vi "PH_Test.vi"() -> ()   [LabVIEW 8.6]
panel:
  out "Router Info":T1(array[cluster])
  out "Range":i32
  out "Resolution (ps)":i32
  out "error out":errorcluster
  out "Library Version":string="2.1"
  in  "error in (no error)":errorcluster
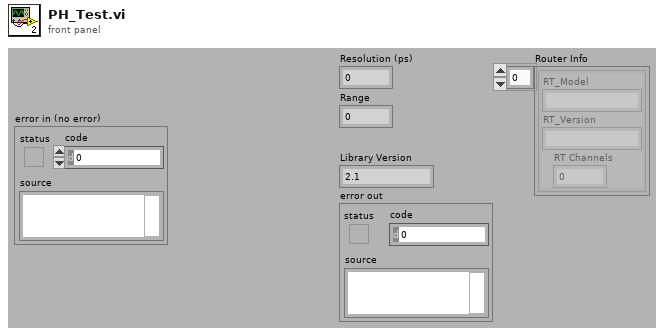
[diagram p1: front panel]
types:
  T1 = cluster{"RT_Model":string, "RT_Version":string, "RT Channels":i32}[]
  T2 = cluster{"Dev":i32, "SerNo":string, "HW_Model":string, "HW_Version":string}[]
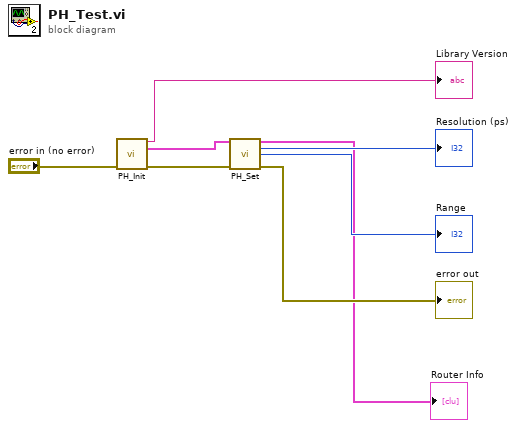
[diagram p0: block diagram]
diagram:
  n1 = call "PH_Init.vi"("error in (no error)"="error in (no error)") -> ("Library Version"=→"Library Version":string, "Device List"=w6:T2, "error out"=w7:errorcluster)  [unwired: 12 in]
  n2 = call "PH_Set.vi"("Device List"=w6, "error in (no error)"=w7) -> ("Router Info"=→"Router Info":T1, "Resolution (ps)"=→"Resolution (ps)":i32, "Range"=→"Range":i32, "error out"=→"error out":errorcluster)  [unwired: 8 in, 2 out]
